vi "Unsimulate.vi"(8 "index":i32, 9 "port":i32(ring) items=["DIN", "DOUT", "RDO", "OPOUT", "TPOUT", "WDI", "WDO", "AIN", "AOUT", "GIN", "GOUT"], 10 "Telnet":refnum<k24>, 11 "error in":errorcluster) -> (0 "ErrorText":string, 1 "Succeed":bool, 2 "KclCommand":string, 3 "error out":errorcluster)   [LabVIEW 2015, in "UnderAutomation.Fanuc.lvlib"]
uses:
  UnderAutomation.Fanuc.lvlib
  C:/Users/fg/Documents/Fanuc.vi/LabVIEW_2024/UnderAutomation.Fanuc/lib/UnderAutomation.Fanuc.dll
  LabVIEW_2024/UnderAutomation.Fanuc/lib/UnderAutomation.Fanuc.dll
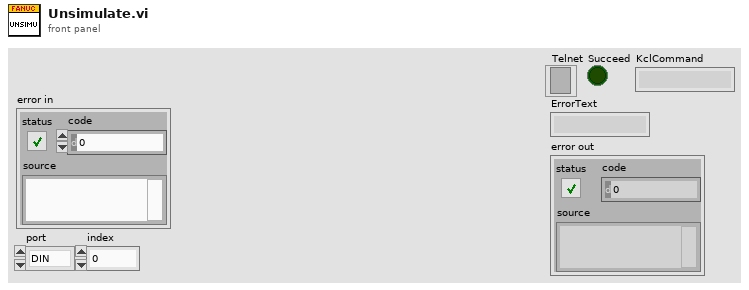
[diagram p1: front panel]
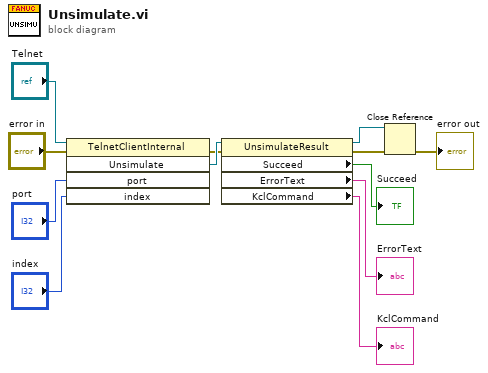
[diagram p0: block diagram]
diagram:
  n1 = invoke class="TelnetClientInternal" method="Unsimulate"(reference="Telnet", error in="error in", "port"="port", "index"="index") -> (error out=w7:errorcluster, "Unsimulate"=w10:refnum<k24>)  [unwired: 1 in, 3 out]
  n2 = property class="UnsimulateResult"(reference=w10, error in=w7) -> (reference out=w3:refnum<k24>, error out=w4:errorcluster, "Succeed"=→"Succeed":bool, "ErrorText"=→"ErrorText":string, "KclCommand"=→"KclCommand":string)
  n3 = Close Reference(reference=w3, error in (no error)=w4) -> (error out=→"error out":errorcluster)
